vi "Ground_Control_Station_V2.vi"() -> ()   [LabVIEW 2014]
panel:
  in  "?":enum32{"Voltage", "Current"}(tab)
  out "Voltage":dbl(graph)
  out "Current":dbl(graph)
  in  "address":string
  out "Flags":string
  out "4":dbl
  out "3":dbl
  out "2":dbl
  out "1":dbl
  out "r dot":dbl
  out "q dot":dbl
  out "p dot":dbl
  out "r":dbl
  out "q":dbl
  out "p":dbl
  out "psi (yaw)":dbl
  out "theta (roll)":dbl
  out "phi (pitch)":dbl
  out "z dot":dbl
  out "y dot":dbl
  out "u dot":dbl
  out "w":dbl
  out "v":dbl
  out "u":dbl
  out "Z":dbl
  out "Y":dbl
  out "X":dbl
  out "Current State":string
  in  "remote port or service name":u16
  in  "?":T1(tab)
  out "Engines":T2(graph)
  out "Engine 1":dbl(graph)
  out "Engine 2":dbl(graph)
  out "Engine 3":dbl(graph)
  out "Engine 4":dbl(graph)
  in  "?":T3(tab)
  out "Overview":T4(graph)
  out "TC 1":dbl(graph)
  out "TC 2":dbl(graph)
  out "TC 3":dbl(graph)
  out "TC 4":dbl(graph)
  out "TC 5":dbl(graph)
  out "TC 6":dbl(graph)
  in  "?":T5(tab)
  out "Overview":T6(graph)
  out "PT 1":dbl(graph)
  out "PT 2":dbl(graph)
  out "PT 3":dbl(graph)
  out "PT 4":dbl(graph)
  out "PT 5":dbl(graph)
  out "PT 6":dbl(graph)
  out "PT 7":dbl(graph)
  out "horizon":picture
  out "Offset":dbl[](array[numeric])
  out "Multiplier":dbl[](array[numeric])
  in  "AV5-T":bool
  in  "AV6-T":bool
  in  "FC-U":bool
  in  "FO-U":bool
  out "AV4-T":bool
  out "AV3-T":bool
  out "AV2-T":bool
  out "AV1-T":bool
  out "AV6-T":bool
  out "AV5-T":bool
  out "FO-U":bool
  out "FC-U":bool
  out "?":dbl(slide) scale=0.2..200.0
  in  "Configure \nGraphs":bool
  # "FC-U"
  # "FO-U"
  # "State Variables"
  # "Thrusts"
  # "AV1-T"
  # "AV2-T"
  # "AV3-T"
  # "AV4-T"
  # "AV5-T"
  # "AV6-T"
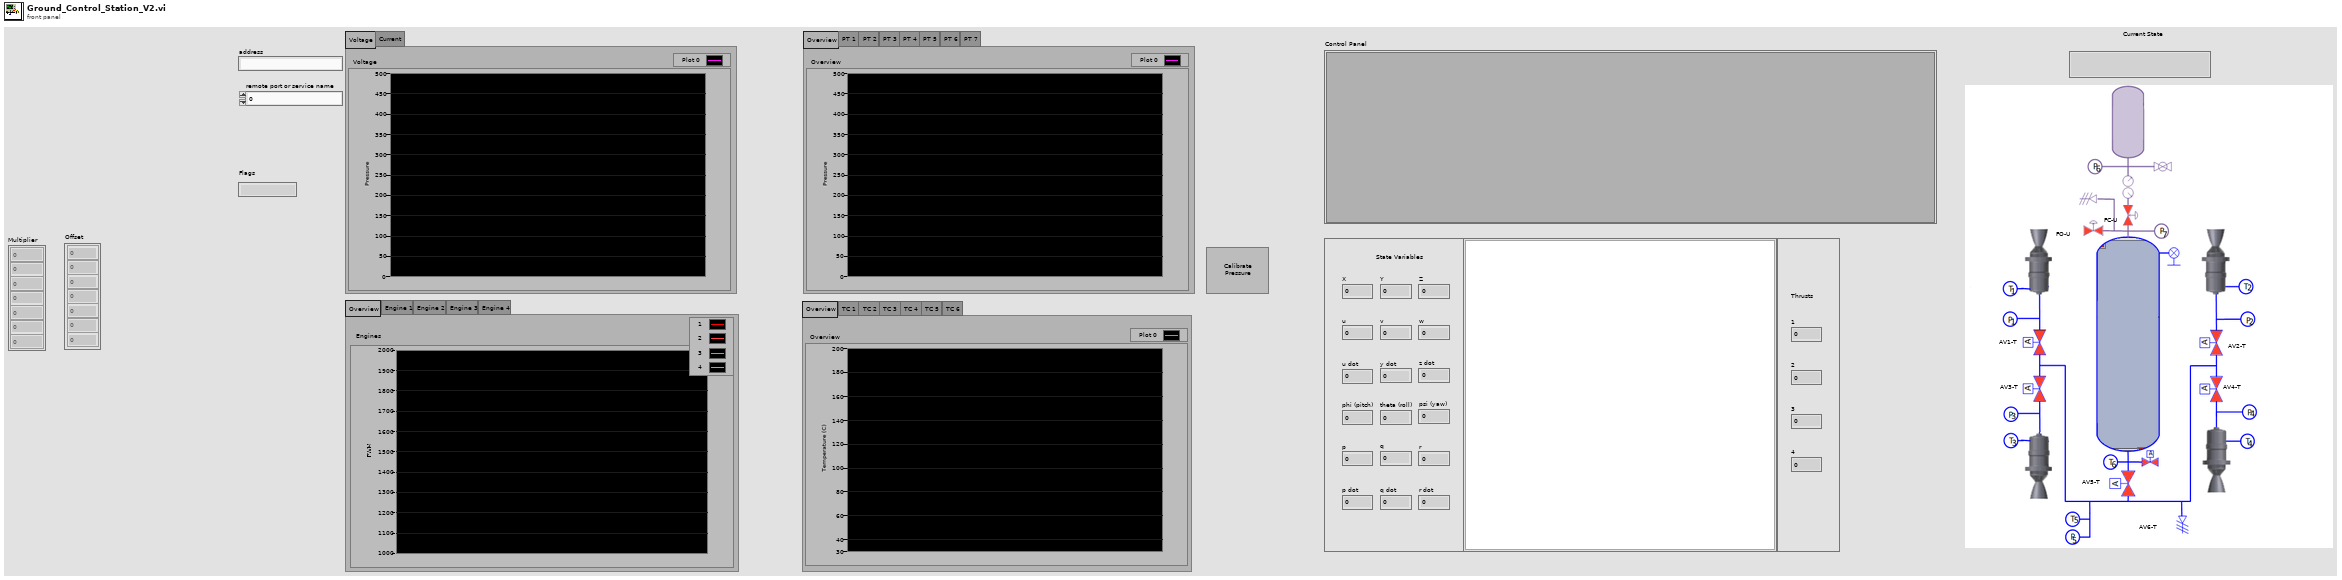
[diagram p1: front panel]
types:
  T1 = enum32{"Overview", "Engine 1", "Engine 2", "Engine 3", "Engine 4"}
  T2 = cluster{"valves[0]":dbl, "valves[1]":dbl, "valves[2]":dbl, "valves[3]":dbl}
  T3 = enum32{"Overview", "TC 1", "TC 2", "TC 3", "TC 4", "TC 5", "TC 6"}
  T4 = cluster{"T Array[0]":dbl, "T Array[1]":dbl, "T Array[2]":dbl, "T Array[3]":dbl, "T Array[4]":dbl, "T Array[5]":dbl}
  T5 = enum32{"Overview", "PT 1", "PT 2", "PT 3", "PT 4", "PT 5", "PT 6", "PT 7"}
  T6 = cluster{"P Array[0]":dbl, "P Array[1]":dbl, "P Array[2]":dbl, "P Array[3]":dbl, "P Array[4]":dbl, "P Array[5]":dbl, "P Array[6]":dbl}
  T7 = enum16{"Standby", "Autonomous", "Position Hold", "Softkill", "Hardkill"}
  T8 = cluster{"thrust[0]":dbl, "thrust[1]":dbl, "thrust[2]":dbl, "thrust[3]":dbl}
  T9 = cluster{"State Variables[0]":dbl, "State Variables[1]":dbl, "State Variables[2]":dbl, "State Variables[3]":dbl, "State Variables[4]":dbl, "State Variables[5]":dbl, "State Variables[6]":dbl, "State Variables[7]":dbl, "State Variables[8]":dbl, "State Variables[9]":dbl, "State Variables[10]":dbl, "State Variables[11]":dbl, "State Variables[12]":dbl, "State Variables[13]":dbl, "State Variables[14]":dbl, "State Variables[15]":dbl, "State Variables[16]":dbl, "State Variables[17]":dbl}
  T10 = cluster{"Electrical[0]":dbl, "Electrical[1]":dbl}
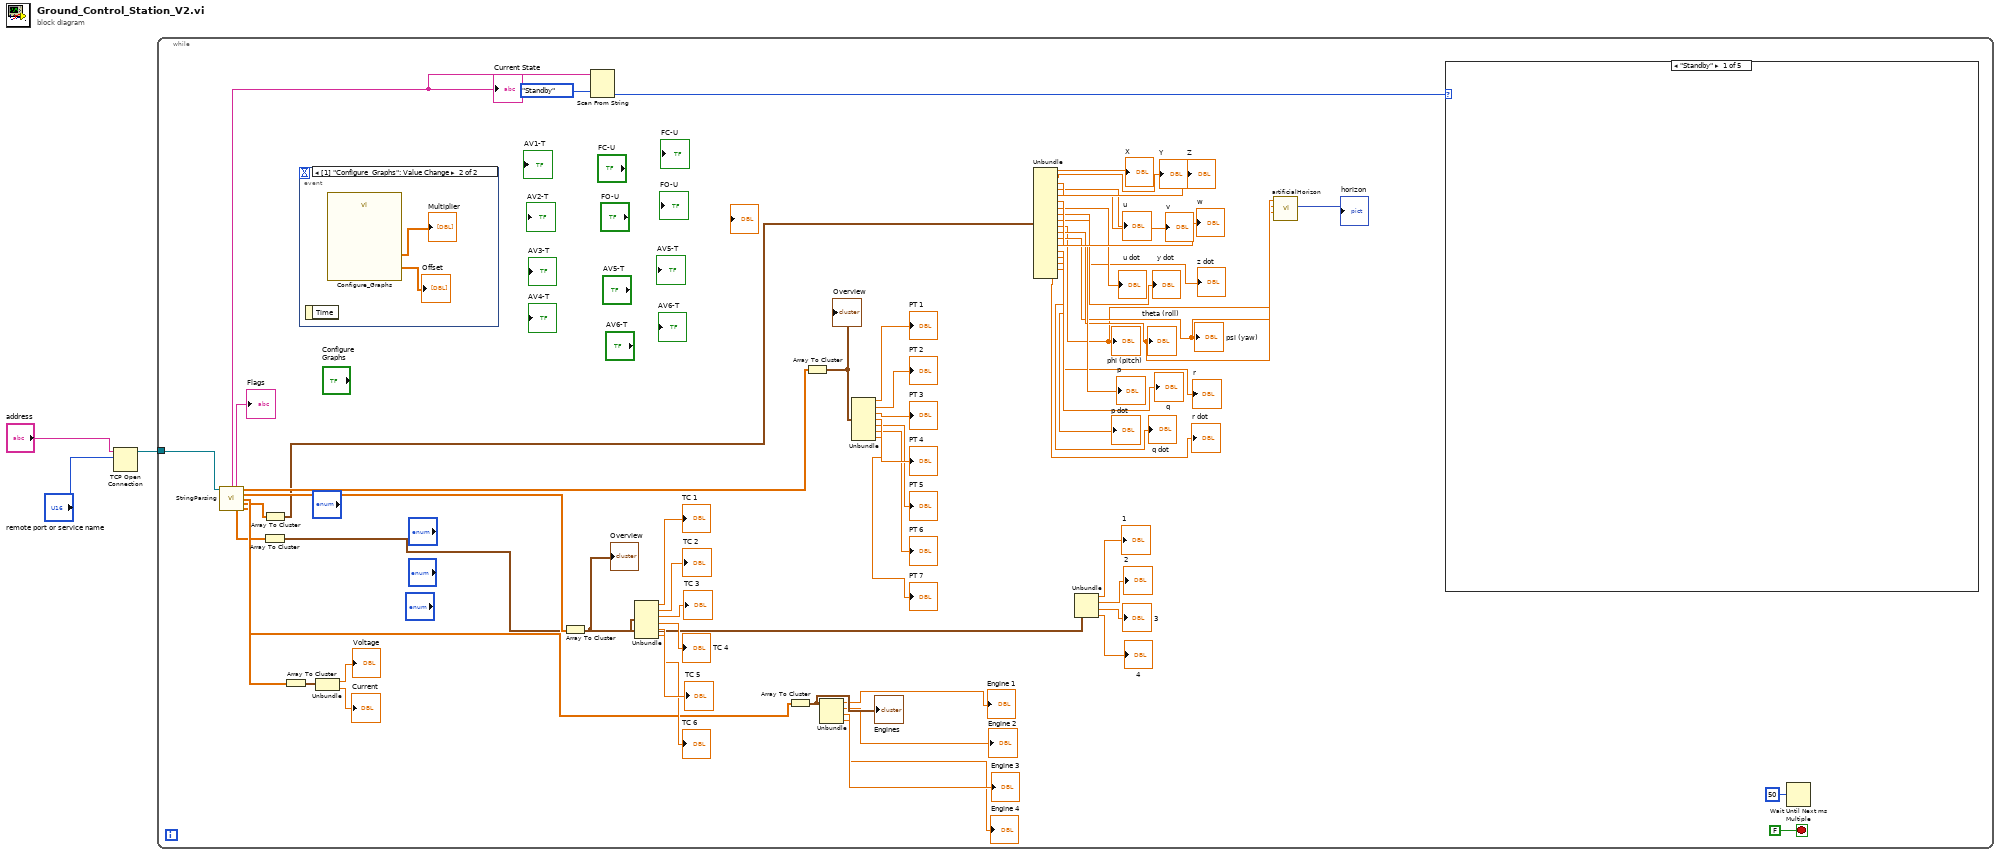
[diagram p0: block diagram]
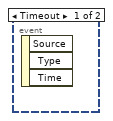
[diagram p2: hidden frame]
diagram:
  n1 = TCP Open Connection(address="address", remote port or service name="remote port or service name") -> (connection ID=w2:refnum<k5>)  [unwired: 3 in, 1 out]
  n2 = while {
    tunnel: w2 -> [w60]
    stop <- FALSE stop-if-true
    n3 = call "StringParsing.vi"("connection ID"=w60) -> ("State"=w58:string, "Flags"=→"Flags":string, "P Array"=w56:dbl[], "T Array"=w47:dbl[], "Electrical"=w39:dbl[], "State Variables"=w29:dbl[], "thrust"=w28:dbl[], "valves"=w34:dbl[])  [unwired: 7 in]
    "Current State" <- w58
    n4 = Array To Cluster(array=w28) -> (cluster=w26:T8)
    n5 = Array To Cluster(array=w29) -> (cluster=w27:T9)
    n6 = Array To Cluster(array=w39) -> (cluster=w38:T10)
    n7 = event shown="[1] \"Configure  Graphs\": Value Change" {
      selector: _ -> [_ _]
      dyn-events: _ -> [_ _]
      timeout: _ -> [_ _]
      event Timeout {
        n8 = event-data() -> ()  [unwired: 1 in, 3 out]
      }
      event "Configure \nGraphs": Value Change {
        n9 = event-data() -> ()  [unwired: 1 in, 1 out]
        n10 = call "Configure_Graphs.vi"() -> ("Output\nMultiple"=→"Multiplier":dbl[], "Output\nOffset"=→"Offset":dbl[])  [unwired: 14 in]
      }
    }
    n11 = Unbundle(w38) -> ("Electrical[0]"=→"Voltage":dbl, "Electrical[1]"=→"Current":dbl)
    n12 = Array To Cluster(array=w47) -> (cluster=w46:T4)
    "Overview" <- w46
    n13 = Scan From String(input string=w58, default 1=T7."Standby") -> (output 1=w61:T7)  [unwired: 3 in, 3 out]
    n14 = Unbundle(w46) -> ("T Array[0]"=→"TC 1":dbl, "T Array[1]"=→"TC 2":dbl, "T Array[2]"=→"TC 3":dbl, "T Array[3]"=→"TC 4":dbl, "T Array[4]"=→"TC 5":dbl, "T Array[5]"=→"TC 6":dbl)
    n15 = Array To Cluster(array=w34) -> (cluster=w35:T2)
    "Engines" <- w35
    n16 = Array To Cluster(array=w56) -> (cluster=w55:T6)
    "Overview" <- w55
    n17 = Unbundle(w35) -> ("valves[0]"=→"Engine 1":dbl, "valves[1]"=→"Engine 2":dbl, "valves[2]"=→"Engine 3":dbl, "valves[3]"=→"Engine 4":dbl)
    n18 = Unbundle(w55) -> ("P Array[0]"=→"PT 1":dbl, "P Array[1]"=→"PT 2":dbl, "P Array[2]"=→"PT 3":dbl, "P Array[3]"=→"PT 4":dbl, "P Array[4]"=→"PT 5":dbl, "P Array[5]"=→"PT 6":dbl, "P Array[6]"=→"PT 7":dbl)
    n19 = Unbundle(w27) -> ("State Variables[0]"=→"X":dbl, "State Variables[1]"=→"Y":dbl, "State Variables[2]"=→"Z":dbl, "State Variables[3]"=→"u":dbl, "State Variables[4]"=→"v":dbl, "State Variables[5]"=→"w":dbl, "State Variables[6]"=→"u dot":dbl, "State Variables[7]"=→"y dot":dbl, "State Variables[8]"=→"z dot":dbl, "State Variables[9]"=w4:dbl, "State Variables[10]"=w6:dbl, "State Variables[11]"=w5:dbl, "State Variables[12]"=→"p":dbl, "State Variables[13]"=→"q":dbl, "State Variables[14]"=→"r":dbl, "State Variables[15]"=→"p dot":dbl, "State Variables[16]"=→"q dot":dbl, "State Variables[17]"=→"r dot":dbl)
    "phi (pitch)" <- w4
    "theta (roll)" <- w6
    "psi (yaw)" <- w5
    n20 = Unbundle(w26) -> ("thrust[0]"=→"1":dbl, "thrust[1]"=→"2":dbl, "thrust[2]"=→"3":dbl, "thrust[3]"=→"4":dbl)
    n21 = call "artificialHorizon.vi"("pitch"=w4, "yaw"=w5, "roll"=w6) -> ("horizon picture"=→"horizon":picture)  [unwired: 8 in]
    n22 = case shown="\"Standby\"" w61 {
      frame "Standby" {
      }
      frame "Autonomous" {
      }
      frame "Position Hold" {
      }
      frame "Softkill" {
      }
      frame "Hardkill" {
      }
    }
    n23 = Wait Until Next ms Multiple(millisecond multiple=u32 50) -> ()  [unwired: 1 out]
  }
